vi "Generate Sweep Pattern.vi"(6 "Sampling":cluster{"Fs":dbl, "#s":i32}, 7 "Sweep Pattern":T1, 8 "error in (no error)":errorcluster, 9 "Sweep Lockin Time (s)":dbl, 10 "Sweep End":dbl, 11 "Sweep Start":dbl) -> (0 "error out":errorcluster, 3 "Sweep Pattern":dbl[](array[numeric]))   [LabVIEW 2019, in "Instrument.DAQ.lvclass"]
uses:
  Instrument.DAQ.lvclass
  Typedefs/Sweep Pattern--Enum.ctl
  <vilib>/Analysis/1siggen.llb/Ramp Pattern by Samples.vi
  <vilib>/Analysis/NI_AALBase.lvlib
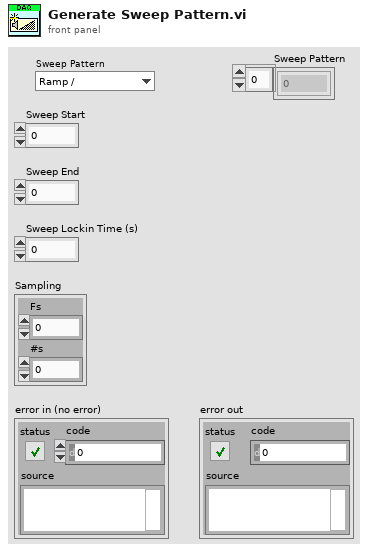
[diagram p1: front panel]
types:
  T1 = typedef "Instrument.DAQ.lvclass/Sweep Pattern--Enum.ctl" = enum16{"Ramp /", "Ramp /\\", "Smooth Ramp _/", "Smooth Ramp _/\\_", "Frequency"}
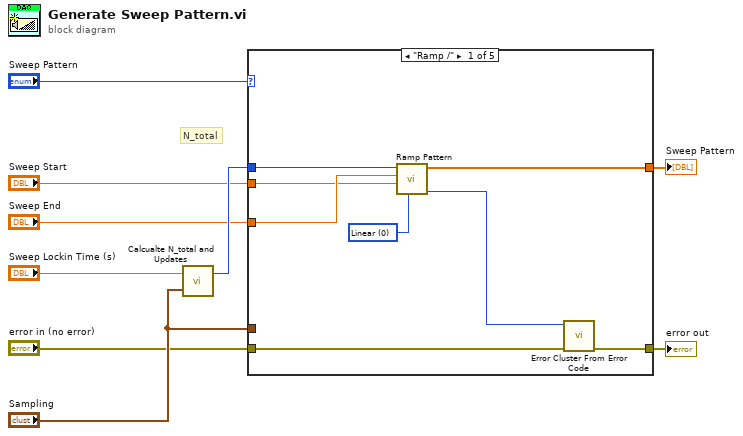
[diagram p0: block diagram]
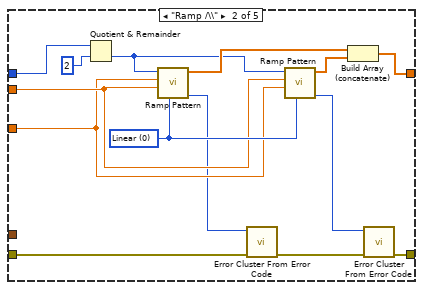
[diagram p2: hidden frame]
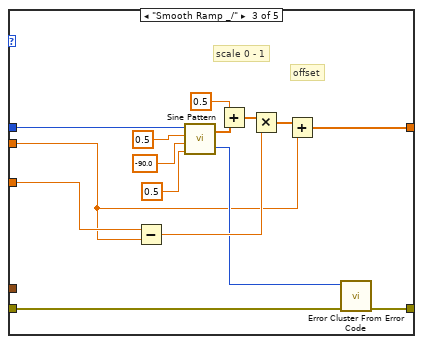
[diagram p3: hidden frame]
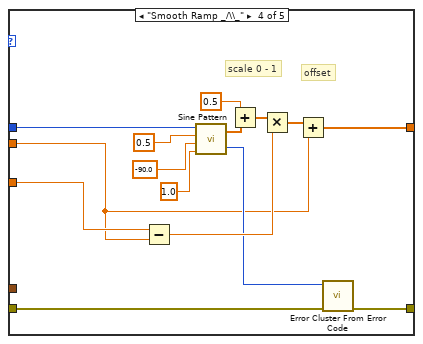
[diagram p4: hidden frame]
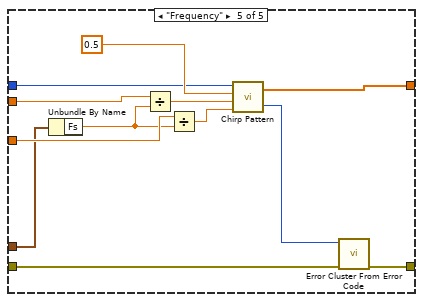
[diagram p5: hidden frame]
diagram:
  # "N_total"
  n1 = call "Calcualte N_total and Updates.vi"("Sampling"="Sampling", "Sweep Time (s)"="Sweep Lockin Time (s)") -> ("N_Total"=w9:i32)  [unwired: 1 out]
  n2 = case shown="\"Ramp /\"" "Sweep Pattern" {
    tunnel: "Sweep End" -> [w15 w25 w46 w61 w72]
    tunnel: "Sweep Start" -> [w14 w26 w33 w49 w68]
    tunnel: [w17 w18 w38 w54 w69] -> w3
    tunnel: [w12 w20 w35 w52 w65] -> w5
    tunnel: "error in (no error)" -> [w13 w22 w36 w51 w66]
    tunnel: w9 -> [w10 w19 w34 w50 w64]
    tunnel: "Sampling" -> [_ _ _ _ w62]
    frame "Ramp /" {
      w16 = u16 0 items=["Linear", "Logarithmic"] ("type")
      n3 = call-poly <vilib>:"Ramp Pattern.vi"("type"=w16, "start"=w14, "end"=w15, "samples"=w10) -> ("error"=w11:i32, "Ramp Pattern"=w17:dbl[])  [unwired: 6 in]
      n4 = call <vilib>:"Error Cluster From Error Code.vi"("error in (no error)"=w13, "error code (0)"=w11) -> ("error out"=w12:errorcluster)  [unwired: 7 in]
    }
    frame "Ramp /\\" {
      w27 = u16 0 items=["Linear", "Logarithmic"] ("type")
      n5 = Quotient & Remainder(x=w19, y=2) -> (floor(x/y)=w29:i32)  [unwired: 1 out]
      n6 = call-poly <vilib>:"Ramp Pattern.vi"("type"=w27, "start"=w26, "end"=w25, "samples"=w29) -> ("error"=w23:i32, "Ramp Pattern"=w31:dbl[])  [unwired: 6 in]
      n7 = call <vilib>:"Error Cluster From Error Code.vi"("error in (no error)"=w22, "error code (0)"=w23) -> ("error out"=w21:errorcluster)  [unwired: 7 in]
      n8 = call-poly <vilib>:"Ramp Pattern.vi"("type"=w27, "start"=w25, "end"=w26, "samples"=w29) -> ("error"=w24:i32, "Ramp Pattern"=w30:dbl[])  [unwired: 6 in]
      n9 = Build Array (concatenate)(w31, w30) -> (w18:dbl[])
      n10 = call <vilib>:"Error Cluster From Error Code.vi"("error in (no error)"=w21, "error code (0)"=w24) -> ("error out"=w20:errorcluster)  [unwired: 7 in]
    }
    frame "Smooth Ramp _/" {
      # "offset"
      # "scale 0 - 1"
      n11 = Subtract(x=w46, y=w33) -> (x-y=w40:dbl)
      n12 = call <vilib>:"Sine Pattern.vi"("cycles"=0.5 ("cycles 2"), "phase(degrees)"=-90.0, "amplitude"=0.5, "samples"=w34) -> ("error"=w37:i32, "Sinusoidal Pattern"=w44:dbl[])
      n13 = Add(x=0.5 ("cycles 2"), y=w44) -> (x+y=w41:dbl[])
      n14 = Multiply(x=w41, y=w40) -> (x*y=w39:dbl[])
      n15 = Add(x=w39, y=w33) -> (x+y=w38:dbl[])
      n16 = call <vilib>:"Error Cluster From Error Code.vi"("error in (no error)"=w36, "error code (0)"=w37) -> ("error out"=w35:errorcluster)  [unwired: 7 in]
    }
    frame "Smooth Ramp _/\\_" {
      # "offset"
      # "scale 0 - 1"
      n17 = Subtract(x=w61, y=w49) -> (x-y=w56:dbl)
      n18 = call <vilib>:"Sine Pattern.vi"("cycles"=1.0 ("cycles 2"), "phase(degrees)"=-90.0, "amplitude"=0.5, "samples"=w50) -> ("error"=w53:i32, "Sinusoidal Pattern"=w59:dbl[])
      n19 = Add(x=0.5 ("cycles 2"), y=w59) -> (x+y=w57:dbl[])
      n20 = Multiply(x=w57, y=w56) -> (x*y=w55:dbl[])
      n21 = Add(x=w55, y=w49) -> (x+y=w54:dbl[])
      n22 = call <vilib>:"Error Cluster From Error Code.vi"("error in (no error)"=w51, "error code (0)"=w53) -> ("error out"=w52:errorcluster)  [unwired: 7 in]
    }
    frame "Frequency" {
      n23 = Unbundle By Name(w62) -> ("Fs"=w63:dbl)
      n24 = Divide(x=w68, y=w63) -> (x/y=w73:dbl)
      n25 = Divide(x=w72, y=w63) -> (x/y=w71:dbl)
      n26 = call <vilib>:"Chirp Pattern.vi"("f2"=w71, "f1"=w73, "amplitude"=0.5, "samples"=w64) -> ("error"=w67:i32, "Chirp Pattern"=w69:dbl[])
      n27 = call <vilib>:"Error Cluster From Error Code.vi"("error in (no error)"=w66, "error code (0)"=w67) -> ("error out"=w65:errorcluster)  [unwired: 7 in]
    }
  }
  "error out" <- w5
  "Sweep Pattern" <- w3
